vi "Go Straight.vi"(2 "Input Right":dbl, 3 "Input Left":dbl) -> (0 "Output Right":dbl, 1 "Output Left":dbl)   [LabVIEW 2013]
uses:
  Robot Global Data.vi
  <vilib>/addons/control/pid/pid.llb/PID (DBL).vi
  <vilib>/addons/control/pid/NI_PID_pid.lvlib
panel:
  in  "PID gains":T1={"proportional gain (Kc)"=0.015, "integral time (Ti, min)"=0.0, "derivative time (Td, min)"=0.0} {"derivative time (Td, min)" format="%.3f"; "integral time (Ti, min)" format="%.3f"; "proportional gain (Kc)" format="%.3f"}
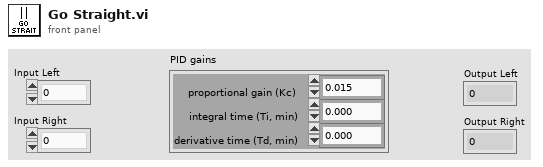
[diagram p1: front panel]
types:
  T1 = cluster{"proportional gain (Kc)":dbl, "integral time (Ti, min)":dbl, "derivative time (Td, min)":dbl}
  T2 = typedef "WPI_GyroDevRef.ctl" = cluster{"DevStatus":errorcluster, "Analog Module":T3, "Analog Channel":T4, "Offset":dbl, "Gain (VoltsPerDegree/Second)":dbl}
  T3 = typedef "FPGA_TypedefAnalogModule.ctl" = enum16{"Analog Module 1", "Analog Module 2"}
  T4 = typedef "FPGA_AIChannel.ctl" = enum8{"AI 1", "AI 2", "AI 3", "AI 4", "AI 5", "AI 6", "AI 7", "AI 8", "Invalid"}
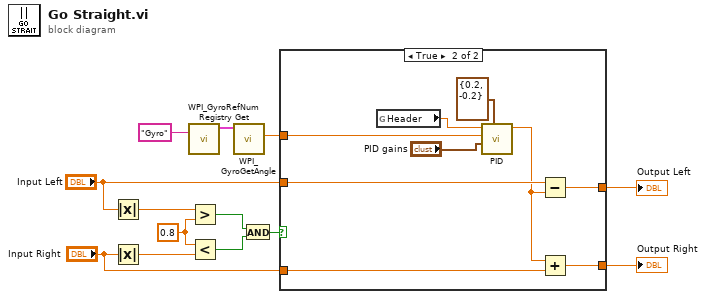
[diagram p0: block diagram]
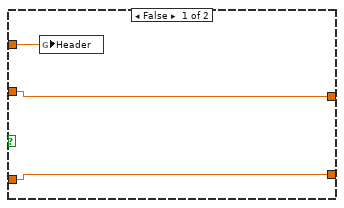
[diagram p2: hidden frame]
diagram:
  w5 = 0.8 ("x")
  n1 = Absolute Value(x="Input Left") -> (abs(x)=w7:dbl)
  n2 = Absolute Value(x="Input Right") -> (abs(x)=w6:dbl)
  n3 = call <vilib>:"WPI_GyroRefNum Registry Get.vi"("refnum name"="Gyro") -> ("GyroDevRef"=w11:T2)  [unwired: 9 in, 1 out]
  n4 = Greater?(x=w7, y=w5) -> (0:w4:bool)
  n5 = Less?(x=w5, y=w6) -> (x < y?=w3:bool)
  n6 = call <vilib>:"WPI_GyroGetAngle.vi"("GyroDevRef"=w11) -> ("Angle"=w10:dbl)  [unwired: 7 in, 3 out]
  n7 = And(x=w4, y=w3) -> (x .and. y?=w9:bool)
  n8 = case shown="True" w9 {
    tunnel: "Input Left" -> [w16 w18]
    tunnel: [w16 w21] -> w13
    tunnel: w10 -> [w15 w25]
    tunnel: [w14 w20] -> w2
    tunnel: "Input Right" -> [w14 w19]
    frame False {
      n9 = global write "Robot Global Data.vi" "Header"(w15) -> ()
    }
    frame True {
      n10 = global read "Robot Global Data.vi" "Header"() -> (w23:dbl)
      n11 = call-poly <vilib>:"PID.vi"("output range"=cluster{"output high":dbl, "output low":dbl} {"output high"=0.2, "output low"=-0.2}, "PID gains"="PID gains", "process variable"=w25, "setpoint"=w23) -> ("output"=w17:dbl)  [unwired: 2 in, 5 out]
      n12 = Subtract(x=w18, y=w17) -> (x-y=w21:dbl)
      n13 = Add(x=w17, y=w19) -> (x+y=w20:dbl)
    }
  }
  "Output Left" <- w13
  "Output Right" <- w2
